vi "Activate.vi"(8 "error in (no error)":errorcluster, 11 "SCADA in":refnum<class "SCADA.lvclass">) -> (0 "error out":errorcluster, 3 "SCADA out":refnum<class "SCADA.lvclass">)   [LabVIEW 2015, in "SCADA Core.lvlib" / "SCADA.lvclass"]
uses:
  SCADA.lvclass
  SCADA.lvclass/SCADA.ctl
  SCADA Messages/Log Msg/Log Msg.lvclass
  SCADA Messages/Measurement Visualization Msg/Measurement Visualization Msg.lvclass
  <vilib>/ActorFramework/Actor/Actor.lvclass/Actor.ctl
  <vilib>/ActorFramework/Message Enqueuer/Message Enqueuer.lvclass/Message Enqueuer.ctl
  IED Actor/IED Messages/PCC Activate Msg/PCC Activate Msg.lvclass/PCC Activate Msg.ctl
  SCADA Abstract Messages/Simple Command Status Msg/Simple Command Status.ctl
  <vilib>/Utility/error.llb/DialogType.ctl
  SCADA Response Messages/Return Activate Status Msg/Return Activate Status Msg.lvclass/Return Activate Status Msg.ctl
  <vilib>/ActorFramework/Message Enqueuer/Init from Existing Queue.vi
  <vilib>/ActorFramework/Message Enqueuer/Enqueue.vi
  <vilib>/ActorFramework/Message Priority Queue/Priority Enqueue.vi
  <vilib>/ActorFramework/Message Enqueuer/Message Enqueuer.lvclass
  IED Actor/IED Messages/PCC Activate Msg/PCC Activate Msg.lvclass
  SCADA Response Messages/Return Activate Status Msg/Return Activate Status Msg.lvclass
  SCADA Abstract Messages/Simple Command Status Msg/Simple Command Status Msg.lvclass
  <vilib>/ActorFramework/Actor/Actor.lvclass
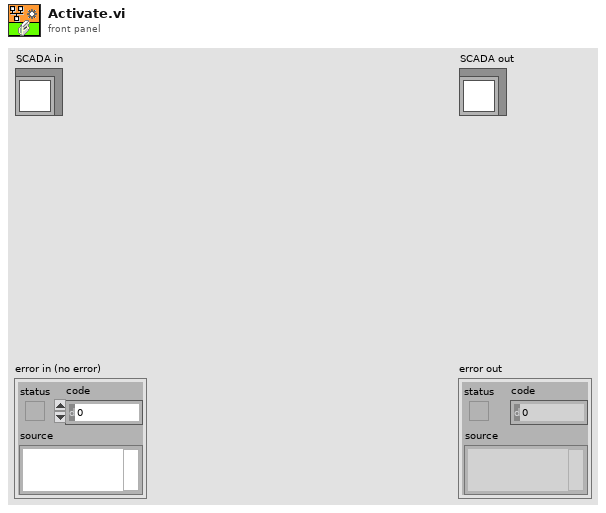
[diagram p1: front panel]
types:
  T1 = typedef "SCADA Core.lvlib/Simple Command Status Msg.lvclass/Simple Command Status.ctl" = enum16{"Success", "Failure"}
  T2 = typedef "SCADA Core.lvlib/SCADA.lvclass/Grid Mode.ctl" = enum16{"Off", "Grid Connected", "Islanded", "Synchronizing"}
  T3 = typedef "DialogType.ctl" = u16
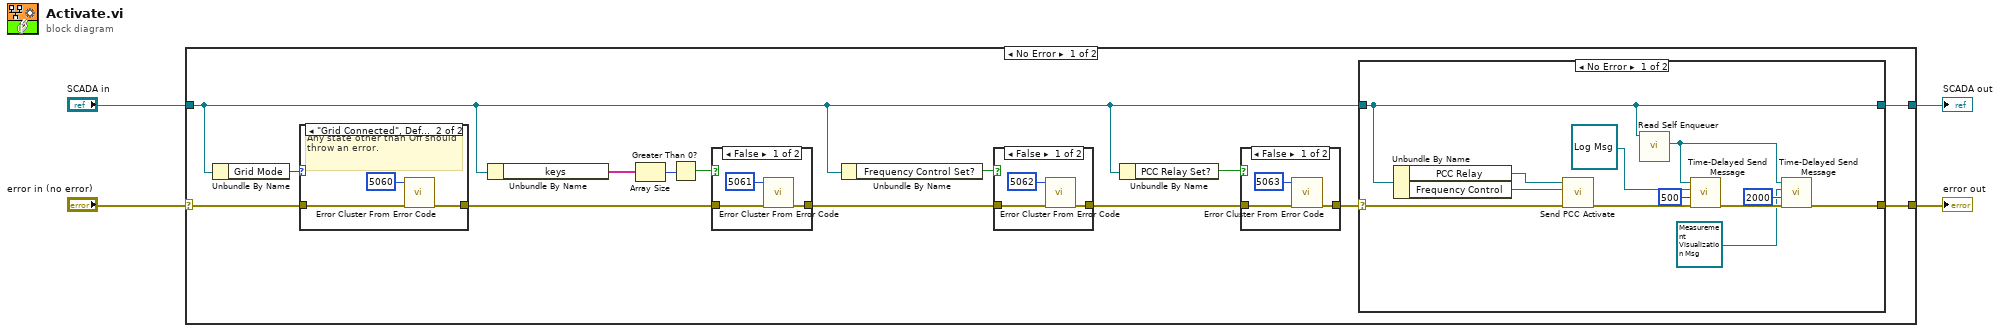
[diagram p0: block diagram]
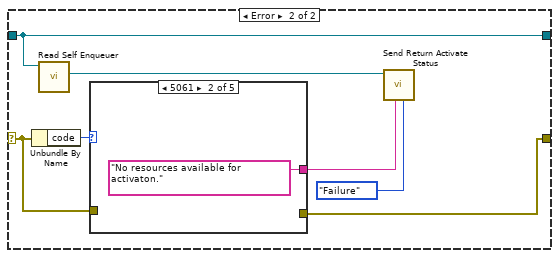
[diagram p2: hidden frame]
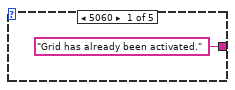
[diagram p3: hidden frame]
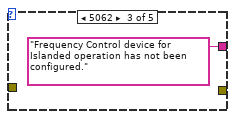
[diagram p4: hidden frame]
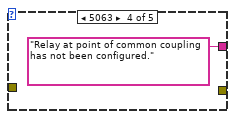
[diagram p5: hidden frame]
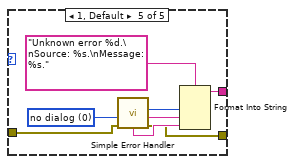
[diagram p6: hidden frame]
diagram:
  n1 = case shown="No Error" "error in (no error)" {
    selector: "error in (no error)" -> [w17 w67]
    tunnel: [w6 w67] -> w3
    tunnel: [w7 w66] -> w1
    tunnel: "SCADA in" -> [w8 w66]
    frame No Error {
      n2 = Unbundle By Name(w8) -> ("Grid Mode"=w18:T2)
      n3 = case shown="\"Grid Connected\", Default" w18 {
        tunnel: w17 -> [w62 w65]
        tunnel: [w62 w63] -> w14
        frame "Off" {
          # "We only want to Activate from the Off state."
        }
        frame "Grid Connected", Default {
          # "Any state other than Off should throw an error."
          n4 = call <vilib>:"Error Cluster From Error Code.vi"("error in (no error)"=w65, "error code (0)"=5060) -> ("error out"=w63:errorcluster)  [unwired: 7 in]
        }
      }
      n5 = Unbundle By Name(w8) -> ("keys"=w16:string[])
      n6 = Array Size(array=w16) -> (size(s)=w15:i32)
      n7 = Greater Than 0?(x=w15) -> (x > 0?=w5:bool)
      n8 = case shown="False" w5 {
        tunnel: w14 -> [w60 w61]
        tunnel: [w58 w61] -> w12
        frame False {
          n9 = call <vilib>:"Error Cluster From Error Code.vi"("error in (no error)"=w60, "error code (0)"=5061) -> ("error out"=w58:errorcluster)  [unwired: 7 in]
        }
        frame True {
        }
      }
      n10 = Unbundle By Name(w8) -> ("Frequency Control Set?"=w13:bool)
      n11 = case shown="False" w13 {
        tunnel: w12 -> [w56 w57]
        tunnel: [w54 w57] -> w10
        frame False {
          n12 = call <vilib>:"Error Cluster From Error Code.vi"("error in (no error)"=w56, "error code (0)"=5062) -> ("error out"=w54:errorcluster)  [unwired: 7 in]
        }
        frame True {
        }
      }
      n13 = Unbundle By Name(w8) -> ("PCC Relay Set?"=w11:bool)
      n14 = case shown="False" w11 {
        tunnel: w10 -> [w52 w53]
        tunnel: [w50 w53] -> w9
        frame False {
          n15 = call <vilib>:"Error Cluster From Error Code.vi"("error in (no error)"=w52, "error code (0)"=5063) -> ("error out"=w50:errorcluster)  [unwired: 7 in]
        }
        frame True {
        }
      }
      n16 = case shown="No Error" w9 {
        selector: w9 -> [w29 w36]
        tunnel: w8 -> [w27 w35]
        tunnel: [w27 w35] -> w7
        tunnel: [w21 w33] -> w6
        frame No Error {
          n17 = Unbundle By Name(w27) -> ("PCC Relay"=w30:refnum<class "Message Enqueuer.lvclass">, "Frequency Control"=w24:refnum<class "Message Enqueuer.lvclass">)
          n18 = call "Send PCC Activate.vi"("error in (no error)"=w29, "Frequency Control"=w24, "Message Enqueuer"=w30) -> ("error out"=w28:errorcluster)  [unwired: 7 in, 1 out]
          n19 = call <vilib>:"Read Self Enqueuer.vi"("Actor"=w27) -> ("Self Enqueuer"=w20:refnum<class "Message Enqueuer.lvclass">)  [unwired: 10 in]
          n20 = call <vilib>:"Time-Delayed Send Message.vi"("error in (no error)"=w28, "Milliseconds To Wait"=500, "Message"=refnum<class "Log Msg.lvclass"> refnum ("SCADA Core.lvlib:Log Msg.lvclass"), "Message Enqueuer"=w20) -> ("error out"=w22:errorcluster)  [unwired: 6 in, 1 out]
          n21 = call <vilib>:"Time-Delayed Send Message.vi"("error in (no error)"=w22, "Milliseconds To Wait"=2000, "Message"=refnum<class "Measurement Visualization Msg.lvclass"> refnum ("SCADA Core.lvlib:Measurement Visualization Msg.lvclass"), "Message Enqueuer"=w20) -> ("error out"=w21:errorcluster)  [unwired: 6 in, 1 out]
        }
        frame Error {
          n22 = Unbundle By Name(w36) -> ("code"=w37:i32)
          n23 = call <vilib>:"Read Self Enqueuer.vi"("Actor"=w35) -> ("Self Enqueuer"=w34:refnum<class "Message Enqueuer.lvclass">)  [unwired: 10 in]
          n24 = case shown="5061" w37 {
            tunnel: w36 -> [_ _ _ _ w44]
            tunnel: ["Grid has already been activated." "No resources available for activaton." "Frequency Control device for Islanded operation has not been configured." "Relay at point of common coupling has not been configured." w43] -> w32
            tunnel: [_ _ _ _ w42] -> w33
            frame 5060 {
            }
            frame 5061 {
            }
            frame 5062 {
            }
            frame 5063 {
            }
            frame 1, Default {
              w45 = T3 0 items=["no dialog", "OK message", "continue or stop message", "OK message + warnings", "continue/stop + warnings"] ("type of dialog (OK msg:1)")
              n25 = call <vilib>:"Simple Error Handler.vi"("type of dialog (OK msg:1)"=w45, "error in (no error)"=w44) -> ("code out"=w47:i32, "source out"=w48:string, "error out"=w42:errorcluster, "message"=w49:string)  [unwired: 3 in, 1 out]
              n26 = Format Into String(format string="Unknown error %d.\nSource: %s.\nMessage: %s." ("Error String"), w47, w48, w49) -> (resulting string=w43:string)  [unwired: 2 in, 1 out]
            }
          }
          n27 = call "Send Return Activate Status.vi"("Status"=Simple_Command_Status."Failure", "error"=w32, "Message Enqueuer"=w34) -> ()  [unwired: 7 in, 2 out]
        }
      }
    }
    frame Error {
    }
  }
  "error out" <- w3
  "SCADA out" <- w1
